vi "Alarma_IEEE45_G06.vi"(8 "error in (no error)":errorcluster) -> (0 "error out":errorcluster)   [LabVIEW 2018]
uses:
  Controls/Cluster_Alarmas_IEEE45.ctl
  <vilib>/RAFA Solutions/Harmony UI Controls Kit/Boolean/Round Led.ctl
  <vilib>/addons/database/Connection.llb/DB Tools Open Connec (Path).vi
  Global/Demo.vi
  Global/Alarmas_indicadores-LED.vi
  Global/AlarmasGlobal.vi
  <vilib>/addons/database/NI_Database_API.lvlib
  <vilib>/RAFA Solutions/Harmony UI Controls Kit/Flat UI Design.lvlib
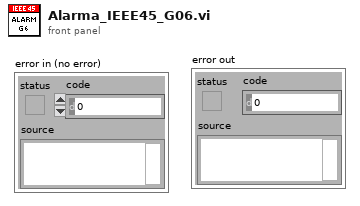
[diagram p1: front panel]
types:
  T1 = typedef "NI_Database_API.lvlib/Conn ObjectReference.ctl" = refnum<k1>
  T2 = typedef "Cluster_Alarmas_IEEE45.ctl" = cluster{"V1_V2 (V) ":cluster{dbl, dbl, dbl}, "Mod_V1_V2":dbl, "alarma 1":T3, "Mod_V2_V3":dbl, "alarma 2":T3, "Mod_V3_V1":dbl, "alarma 3":T3, "Mod_Frec":dbl, "alarma 4":T3, "V2_V3 (V)":cluster{dbl, dbl, dbl}, "V3_V1 (V)":cluster{dbl, dbl, dbl}, "Frecuencia (Hz)":cluster{dbl, dbl, dbl}, "AVG VL_VL (V)":cluster{dbl, dbl, dbl}, "alarm 5":bool, "alarm 6":bool, "alarm 7":bool, "alarm 8":bool, "alarm 9":bool}
  T3 = typedef "Flat UI Design.lvlib/Round Led.ctl" = bool
  T4 = typedef "VIF_cluster.ctl" = cluster{"VL_VL":cluster{"V1_V2":sgl, "V2_V3":sgl, "V3_V1":sgl, "Avg_VL_VL":sgl}, "IL_IL":cluster{"I1":sgl, "I2":sgl, "I3":sgl, "Avg_Amps":sgl}, "Frecuency":sgl, "Avg_Frecuency":sgl}
  T5 = cluster{"V1_V2":sgl, "V2_V3":sgl, "V3_V1":sgl, "Avg_VL_VL":sgl}
  T6 = cluster{"Mod_V1_V2":sgl, "Mod_V2_V3":sgl, "Mod_V3_V1":sgl, "alarma 1":bool, "alarma 2":bool, "alarma 3":bool}
  T7 = cluster{"alarm 5":bool, "alarm 6":bool, "alarm 7":bool, "alarm 8":bool, "alarm 9":bool}
  T8 = cluster{"Frecuency Modulation (%)":sgl, "alarma":bool}
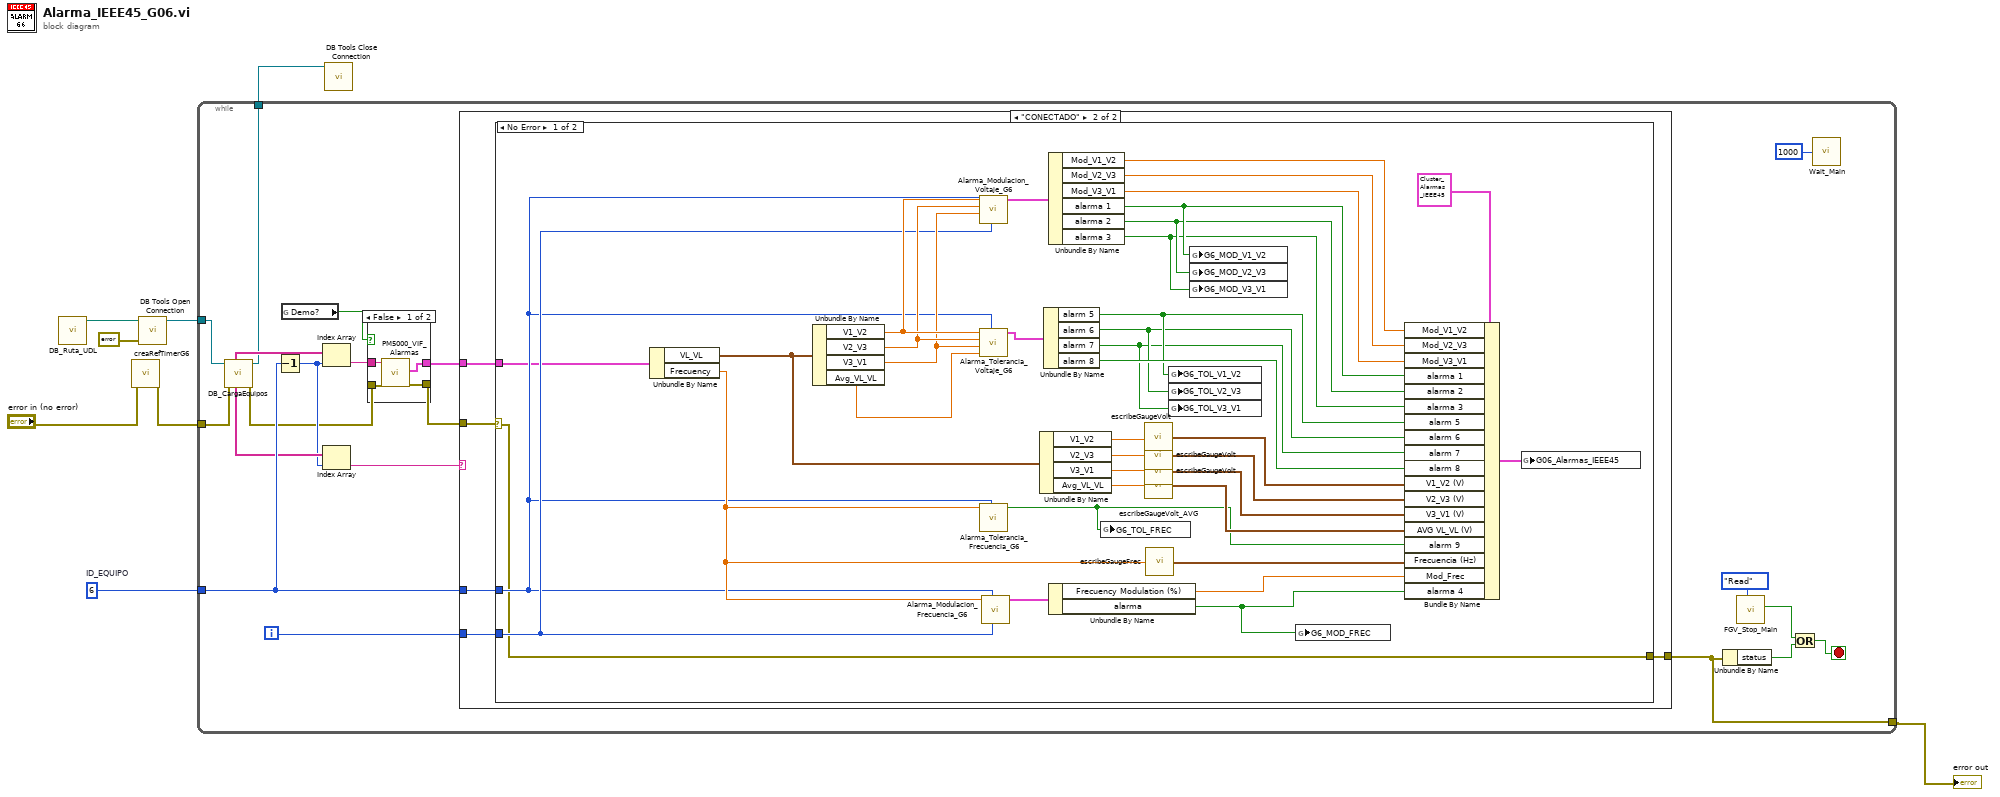
[diagram p0: block diagram]
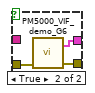
[diagram p2: hidden frame]
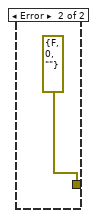
[diagram p4: hidden frame]
diagram:
  w5 = 6  # ID_EQUIPO
  n1 = call "DB_Ruta_UDL.vi"() -> ("UDL ruta"=w3:path)  [unwired: 11 in]
  n2 = call "creaRefTimerG6.vi"("error in (no error)"="error in (no error)") -> ("error out"=w7:errorcluster)  [unwired: 10 in]
  n3 = call-poly <vilib>:"DB Tools Open Connection.vi"("error in (no error)"=errorcluster {"status"=FALSE, "code"=0, "source"=""}, "connection information"=w3) -> ("connection reference"=w2:T1)  [unwired: 6 in, 1 out]
  n4 = while {
    tunnel: w7 -> [w20]
    tunnel: [w22] -> w6
    tunnel: w5 -> [w17]
    tunnel: w2 -> [w19]
    tunnel: [w18] -> w1
    i -> [w26]
    stop <- w25 stop-if-true
    n5 = call "DB_CargaEquipos.vi"("error in (no error)"=w20, "db in"=w19) -> ("error out"=w12:errorcluster, "db out"=w18:T1, "ESTADO_EQUIPO"=w16:string[], "IP_EQUIPOS"=w21:string[])  [unwired: 2 in, 4 out]
    n6 = Decrement(x=w17) -> (x-1=w15:i32)
    n7 = global read "Demo.vi" "Demo?"() -> (w9:bool)
    n8 = Index Array(array=w21, index=w15) -> (element=w13:string)
    n9 = Index Array(array=w16, index=w15) -> (element=w14:string)
    n10 = case shown="False" w9 {
      tunnel: w13 -> [w32 _]
      tunnel: w12 -> [w31 w35]
      tunnel: [w30 w34] -> w11
      tunnel: [w29 w33] -> w10
      frame False {
        n11 = call "PM5000_VIF_Alarmas.vi"("error in"=w31, "Network Path"=w32) -> ("error out"=w30:errorcluster, "output cluster"=w29:T4)  [unwired: 7 in, 1 out]
      }
      frame True {
        n12 = call "PM5000_VIF_demo_G6.vi"("error in (no error)"=w35) -> ("error out"=w34:errorcluster, "VIF_cluster"=w33:T4)  [unwired: 1 in]
      }
    }
    n13 = case shown="\"CONECTADO\"" w14 {
      tunnel: w26 -> [_ w40]
      tunnel: [_ w39] -> w22
      tunnel: w17 -> [_ w38]
      tunnel: w11 -> [_ w37]
      tunnel: w10 -> [_ w36]
      frame Default {
      }
      frame "CONECTADO" {
        n14 = case shown="No Error" w37 {
          selector: w37 -> [w52 _]
          tunnel: w40 -> [w67 _]
          tunnel: [w52 errorcluster {"status"=FALSE, "code"=0, "source"=""} ("error out")] -> w39
          tunnel: w38 -> [w53 _]
          tunnel: w36 -> [w51 _]
          frame No Error {
            n15 = Unbundle By Name(w51) -> ("VL_VL"=w72:T5, "Frecuency"=w66:sgl)
            n16 = Unbundle By Name(w72) -> ("V1_V2"=w77:sgl, "V2_V3"=w76:sgl, "V3_V1"=w75:sgl, "Avg_VL_VL"=w74:sgl)
            n17 = call "Alarma_Modulacion_Voltaje_G6.vi"("# iteration"=w67, "ID_EQUIPO"=w53, "V3_V1"=w75, "V2_V3"=w76, "V1_V2"=w77) -> ("Alarma_Mod_Volt out"=w73:T6)  [unwired: 6 in]
            n18 = call "Alarma_Tolerancia_Voltaje_G6.vi"("ID_EQUIPO"=w53, "AVG_VL_VL"=w74, "V3_V1"=w75, "V2_V3"=w76, "V1_V2"=w77) -> ("alarm out"=w64:T7)  [unwired: 6 in]
            n19 = call "Alarma_Tolerancia_Frecuencia_G6.vi"("ID_EQUIPO"=w53, "Señal in"=w66) -> ("alarm"=w42:bool)  [unwired: 9 in]
            n20 = call "Alarma_Modulacion_Frecuencia_G6.vi"("# iteration"=w67, "ID_EQUIPO"=w53, "Frecuencia"=w66) -> ("Mod_Frec out"=w65:T8)  [unwired: 8 in]
            n21 = Unbundle By Name(w72) -> ("V1_V2"=w71:sgl, "V2_V3"=w70:sgl, "V3_V1"=w69:sgl, "Avg_VL_VL"=w68:sgl)
            n22 = Unbundle By Name(w64) -> ("alarm 5"=w45:bool, "alarm 6"=w44:bool, "alarm 7"=w43:bool, "alarm 8"=w60:bool)
            n23 = Unbundle By Name(w73) -> ("Mod_V1_V2"=w63:sgl, "Mod_V2_V3"=w62:sgl, "Mod_V3_V1"=w61:sgl, "alarma 1"=w48:bool, "alarma 2"=w47:bool, "alarma 3"=w46:bool)
            n24 = Unbundle By Name(w65) -> ("Frecuency Modulation (%)"=w54:sgl, "alarma"=w41:bool)
            n25 = global write "Alarmas_indicadores-LED.vi" "G6_TOL_FREC"(w42) -> ()
            n26 = call "escribeGaugeVolt.vi"("Vin"=w71) -> ("V_V out"=w59:cluster{"Max":sgl, "Vin":sgl, "Min":sgl})
            n27 = call "escribeGaugeVolt.vi"("Vin"=w70) -> ("V_V out"=w58:cluster{"Max":sgl, "Vin":sgl, "Min":sgl})
            n28 = call "escribeGaugeVolt.vi"("Vin"=w69) -> ("V_V out"=w57:cluster{"Max":sgl, "Vin":sgl, "Min":sgl})
            n29 = call "escribeGaugeVolt_AVG.vi"("Vin"=w68) -> ("V_V out"=w56:cluster{"Max":sgl, "Vin":sgl, "Min":sgl})
            n30 = call "escribeGaugeFrec.vi"("Fin"=w66) -> ("Frec out"=w55:cluster{"Max":sgl, "Vin":sgl, "Min":sgl})
            n31 = global write "Alarmas_indicadores-LED.vi" "G6_TOL_V1_V2"(w45) -> ()
            n32 = global write "Alarmas_indicadores-LED.vi" "G6_TOL_V2_V3"(w44) -> ()
            n33 = global write "Alarmas_indicadores-LED.vi" "G6_TOL_V3_V1"(w43) -> ()
            n34 = global write "Alarmas_indicadores-LED.vi" "G6_MOD_V1_V2"(w48) -> ()
            n35 = global write "Alarmas_indicadores-LED.vi" "G6_MOD_V2_V3"(w47) -> ()
            n36 = global write "Alarmas_indicadores-LED.vi" "G6_MOD_V3_V1"(w46) -> ()
            n37 = global write "Alarmas_indicadores-LED.vi" "G6_MOD_FREC"(w41) -> ()
            n38 = Bundle By Name(cluster=T2 {"V1_V2 (V) "={0.0, 17.0, 16.662651515468255}, "Mod_V1_V2"=0.0, "alarma 1"=FALSE, "Mod_V2_V3"=0.0, "alarma 2"=FALSE, "Mod_V3_V1"=0.0, "alarma 3"=FALSE, "Mod_Frec"=0.0, "alarma 4"=FALSE, "V2_V3 (V)"={0.0, 17.0, 16.662651515468255}, "V3_V1 (V)"={0.0, 17.0, 16.662651515468255}, "Frecuencia (Hz)"={0.0, 17.0, 16.662651515468255}, "AVG VL_VL (V)"={0.0, 17.0, 16.662651515468255}, "alarm 5"=FALSE, "alarm 6"=FALSE, "alarm 7"=FALSE, "alarm 8"=FALSE, "alarm 9"=FALSE} ("G06_Alarmas_IEEE45"), "Mod_V1_V2"=w63, "Mod_V2_V3"=w62, "Mod_V3_V1"=w61, "alarma 1"=w48, "alarma 2"=w47, "alarma 3"=w46, "alarm 5"=w45, "alarm 6"=w44, "alarm 7"=w43, "alarm 8"=w60, "V1_V2 (V)"=w59, "V2_V3 (V)"=w58, "V3_V1 (V)"=w57, "AVG VL_VL (V)"=w56, "alarm 9"=w42, "Frecuencia (Hz)"=w55, "Mod_Frec"=w54, "alarma 4"=w41) -> (w49:T2)
            n39 = global write "AlarmasGlobal.vi" "G06_Alarmas_IEEE45"(w49) -> ()
          }
          frame Error {
          }
        }
      }
    }
    n40 = Unbundle By Name(w22) -> ("status"=w23:bool)
    n41 = call "FGV_Stop_Main.vi"("Action"=enum16{"Read", "Write"}."Read") -> ("Var Out"=w24:bool)  [unwired: 9 in, 1 out]
    n42 = Or(x=w24, y=w23) -> (x .or. y?=w25:bool)
    n43 = call "Wait_Main.vi"("Wait time (msec)"=u32 1000 ("delay (ms)")) -> ()  [unwired: 5 in]
  }
  "error out" <- w6
  n44 = call <vilib>:"DB Tools Close Connection.vi"("connection reference"=w1) -> ()  [unwired: 6 in, 1 out]
